vi "configure resonance.vi"(6 "x resonant zoom voltage":dbl, 8 "error in":errorcluster, 10 "Start Delay (Ticks)":i16) -> (0 "bitfile name":T1, 1 "pixels per frame":dbl, 2 "FPGA VI Reference Out":T2, 4 "Actual Depth 3":u32)   [LabVIEW 2012]
doc: "SciScan 1.0 151216"
uses:
  Custom Controls/FPGA reference typedef for 120MHz code.ctl
  Custom Controls/biotfile select.ctl
  Custom Controls/Pockels data structure (for laser power control).ctl
  <vilib>/DAQmx/write.llb/DAQmx Write (Analog DBL 1Chan 1Samp).vi
  <vilib>/DAQmx/write.llb/DAQmx Write (Analog 2D DBL NChan NSamp).vi
  <vilib>/DAQmx/write.llb/DAQmx Write (Analog 1D DBL 1Chan NSamp).vi
  GFG/GFGstringGet.vi
  GFG/GFGbooleanGet.vi
  <vilib>/DAQmx/create/channels.llb/DAQmx Create Channel (AO-Voltage-Basic).vi
  <vilib>/DAQmx/miscellaneous.llb/DAQmx Fill In Error Info.vi
  GFG/GFGnumericGet.vi
  <vilib>/DAQmx/configure/trigger.llb/DAQmx Start Trigger (Digital Edge).vi
  <vilib>/Utility/error.llb/Error Cluster From Error Code.vi
  <vilib>/rvi/errors/niLvFpgaAdjustHostInterfaceError.vi
  <vilib>/rvi/interface/nirviMethod/nirviMethod.xnode
  GFG/GFG library.lvlib
  <resource>/objmgr/daqmx.rc
  <vilib>/rvi/errors/niLvFpgaMergeErrorWithErrorCode.vi
  <vilib>/FPGAPlugInAG/Dynamic/niLvFpga_ReadFifo_Dynamic.vi
panel:
  out "size(s)":i32[](array[numeric])
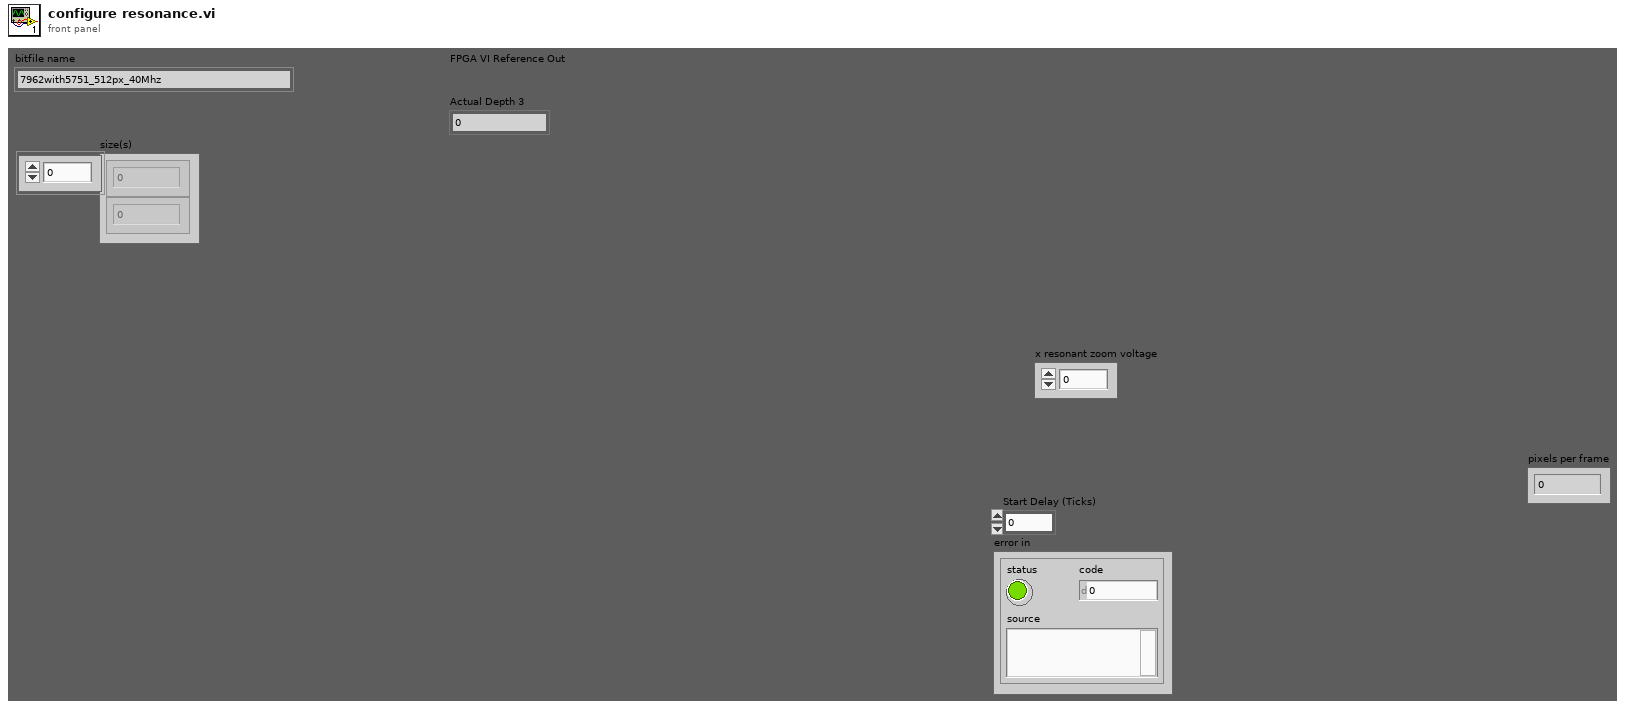
[diagram p1: front panel]
types:
  T1 = typedef "biotfile select.ctl" = enum16{"7962with5751_512px_40Mhz", "7962with5751_512px_50Mhz", "7961with5734_1024px_120Mhz or ext lasersync", "7962with5734_1024px_120Mhz or ext lasersync", "7962with5734_512px_120Mhz or ext lasersync", "7961with5734_512px_120Mhz or ext lasersync", "7962with5751_12kHz_512px_50MHz_4ch", "7962with5751_1536px_2ch_40Mhz", "7962with5751_1536px_2ch_50Mhz", "7962with5751_12kHz_1024px_2ch_50MHz"}
  T2 = typedef "FPGA reference typedef for 120MHz code.ctl" = refnum<k20>
  T3 = typedef "Pockels data structure (for laser power control).ctl" = cluster{"DAQmx Task Name (Pockels)":refnum<k21>, "(Sharing Pocekls Card?)YGalvo, Pockels,Piezo":bool[]}
  T4 = cluster{"bitfile name":T1, dbl, "lasersync enable":bool}
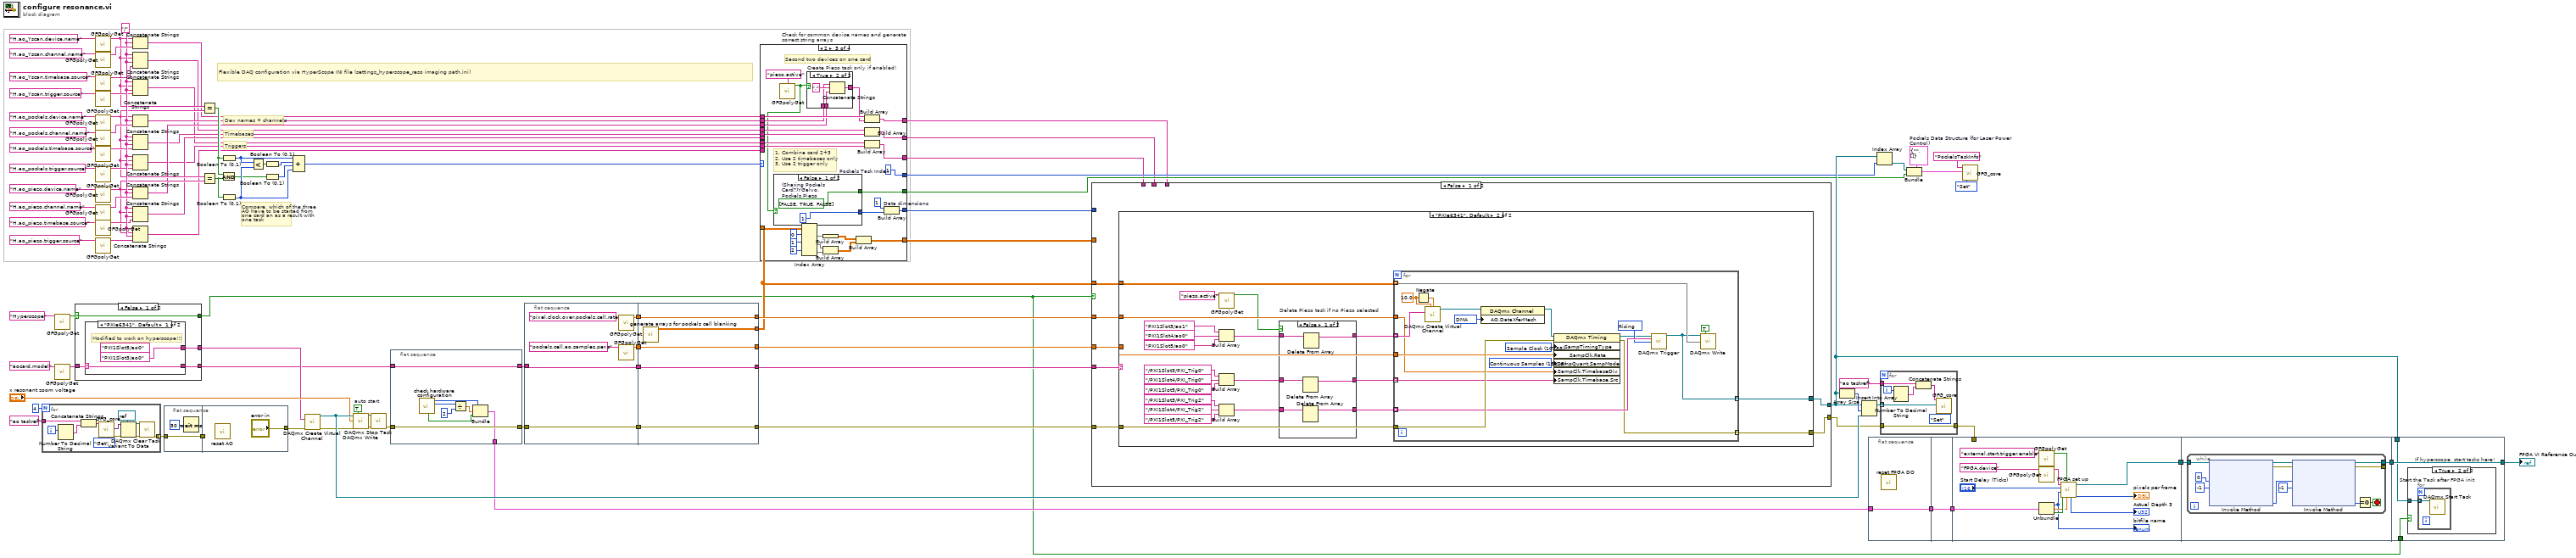
[diagram p0: block diagram]
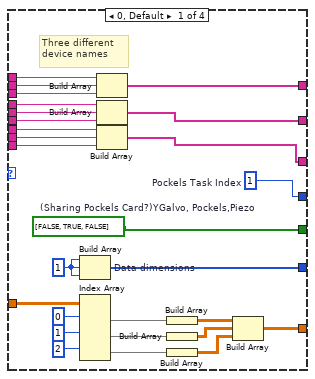
[diagram p2: hidden frame]
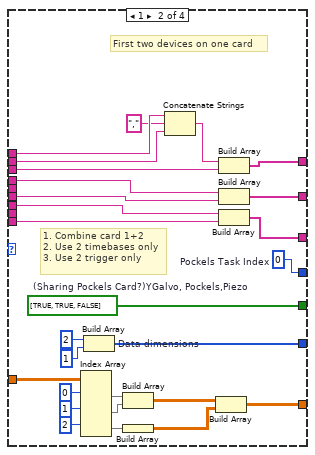
[diagram p3: hidden frame]
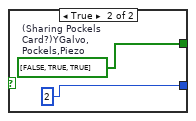
[diagram p4: hidden frame]
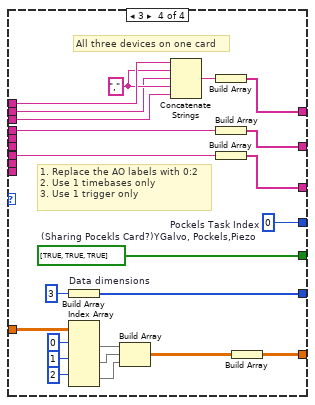
[diagram p6: hidden frame]
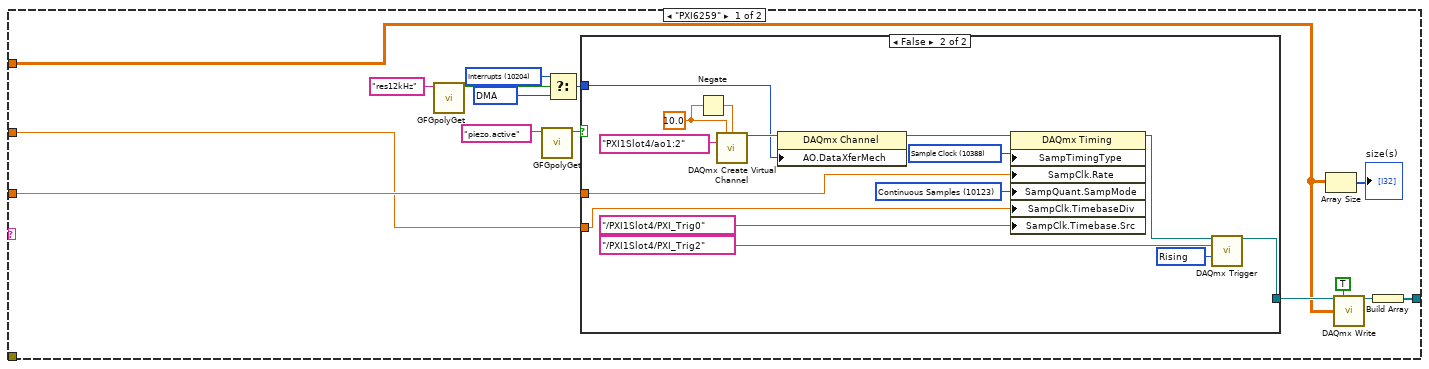
[diagram p7: hidden frame]
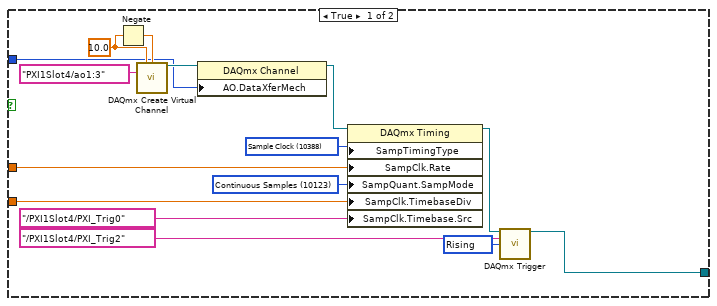
[diagram p8: hidden frame]
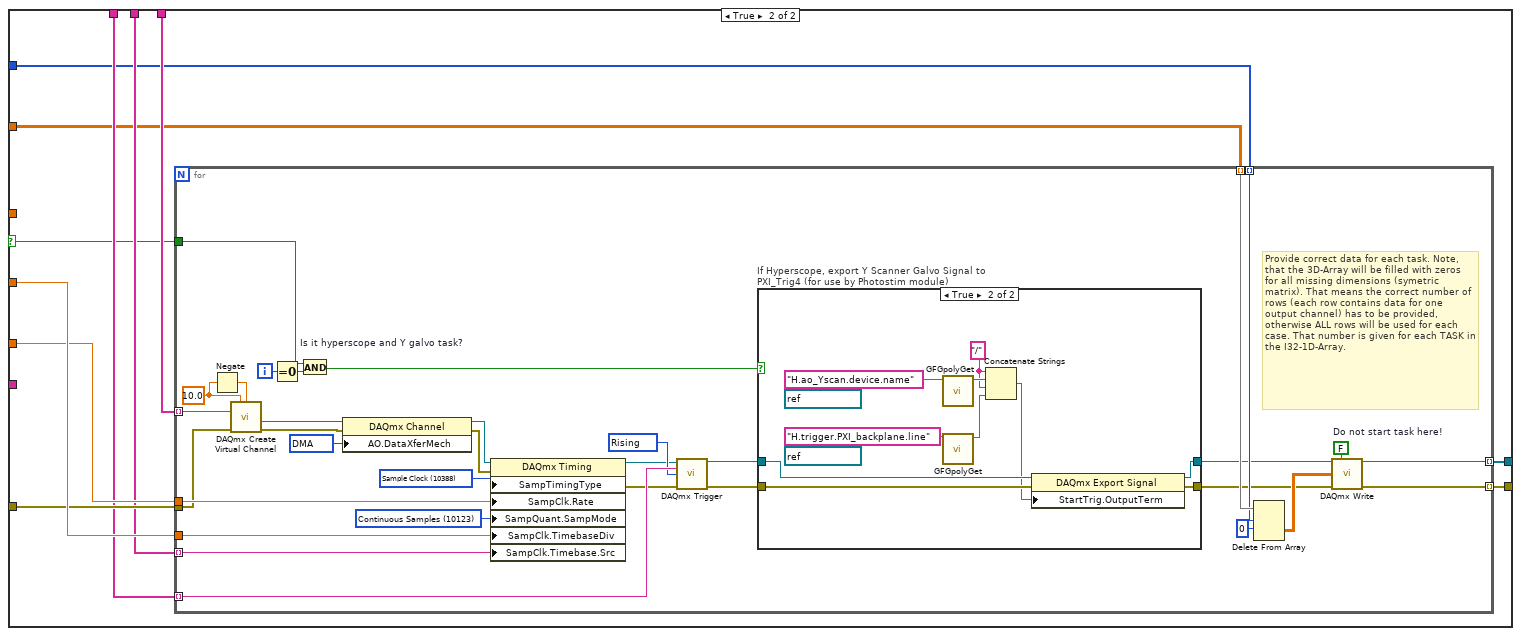
[diagram p10: hidden frame]
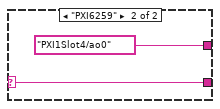
[diagram p12: hidden frame]
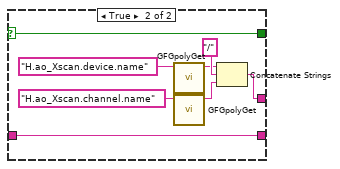
[diagram p13: hidden frame]
diagram:
  w10 = T3 {"DAQmx Task Name (Pockels)"="", "(Sharing Pocekls Card?)YGalvo, Pockels,Piezo"=[]}  # Pockels Data Structure (for Laser Power Control)
  w55 = "/" ("string")
  w91 = TRUE  # auto start
  # "Flexible DAQ configuration via HyperScope INI file (settings_hyperscope_reso imaging path.ini)"
  # "Triggers"
  # "Timebases"
  # "Dev names + channels"
  # "Compare, which of the three AO have to be started from one card an as a result with one task"
  n1 = for {
    N: 4 -> [_]
    tunnel: "ao taskref" ("Variable Name in") -> [w105]
    tunnel: [w100] -> w67 mode=indexing
    i -> [w107]
    n2 = Number To Decimal String(number=w107) -> (decimal integer string=w106:string)  [unwired: 1 in]
    n3 = Concatenate Strings(w105, w106) -> (w104:string)
    n4 = call "GFG_core.vi"("Variable Name in"=w104, "Action"=enum16{"Init", "Set", "Get"}."Get") -> ("Variant Out"=w102:variant, "error out"=w103:errorcluster)  [unwired: 11 in, 5 out]
    n5 = Variant To Data(error in=w103, type=refnum<k21> refnum ("task out"), Variant=w102) -> (data=w99:refnum<k21>, error out=w98:errorcluster)
    n6 = call <vilib>:"DAQmx Clear Task.vi"("task in"=w99, "error in"=w98) -> ("error out"=w100:errorcluster)  [unwired: 13 in]
  }
  n7 = call-poly "GFGpolyGet.vi"("Variable Name in"="aocard.model") -> ("String"=w14:string)  [unwired: 9 in, 1 out]
  n8 = call-poly "GFGpolyGet.vi"("Variable Name in"="Hyperscope") -> ("Boolean Value OUT"=w15:bool)  [unwired: 9 in, 1 out]
  n9 = case shown="False" w15 {
    selector: w15 -> [w110 w118]
    tunnel: [w112 w121] -> w72
    tunnel: w14 -> [w111 w117]
    tunnel: [w110 w118] -> w4
    tunnel: [w109 w117] -> w13
    frame False {
      n10 = case shown="\"PXIe6341\", Default" w111 {
        selector: w111 -> [w114 w115]
        tunnel: [tag "PXI1Slot3/ao0" ("physical channels") tag "PXI1Slot4/ao0" ("physical channels")] -> w112
        tunnel: [w114 w115] -> w109
        frame "PXIe6341", Default {
          (unwired) tag "PXI1Slot5/ao0" ("physical channels")
          # "Modified to work on hyperscope!!!"
        }
        frame "PXI6259" {
        }
      }
    }
    frame True {
      n11 = call-poly "GFGpolyGet.vi"("Variable Name in"="H.ao_Xscan.device.name") -> ("String"=w119:string)  [unwired: 9 in, 1 out]
      n12 = call-poly "GFGpolyGet.vi"("Variable Name in"="H.ao_Xscan.channel.name") -> ("String"=w122:string)  [unwired: 9 in, 1 out]
      n13 = Concatenate Strings(w119, "/" ("String_Output"), w122) -> (w121:string)
    }
  }
  n14 = call-poly "GFGpolyGet.vi"("Variable Name in"="H.ao_Yscan.device.name") -> ("String"=w42:string)  [unwired: 9 in, 1 out]
  n15 = call-poly "GFGpolyGet.vi"("Variable Name in"="H.ao_Yscan.channel.name") -> ("String"=w58:string)  [unwired: 9 in, 1 out]
  n16 = call-poly "GFGpolyGet.vi"("Variable Name in"="H.ao_Yscan.timebase.source") -> ("String"=w52:string)  [unwired: 9 in, 1 out]
  n17 = call-poly "GFGpolyGet.vi"("Variable Name in"="H.ao_Yscan.trigger.source") -> ("String"=w51:string)  [unwired: 9 in, 1 out]
  n18 = call-poly "GFGpolyGet.vi"("Variable Name in"="H.ao_pockels.device.name") -> ("String"=w40:string)  [unwired: 9 in, 1 out]
  n19 = call-poly "GFGpolyGet.vi"("Variable Name in"="H.ao_pockels.channel.name") -> ("String"=w57:string)  [unwired: 9 in, 1 out]
  n20 = call-poly "GFGpolyGet.vi"("Variable Name in"="H.ao_pockels.timebase.source") -> ("String"=w46:string)  [unwired: 9 in, 1 out]
  n21 = call-poly "GFGpolyGet.vi"("Variable Name in"="H.ao_pockels.trigger.source") -> ("String"=w45:string)  [unwired: 9 in, 1 out]
  n22 = call-poly "GFGpolyGet.vi"("Variable Name in"="H.ao_piezo.device.name") -> ("String"=w41:string)  [unwired: 9 in, 1 out]
  n23 = call-poly "GFGpolyGet.vi"("Variable Name in"="H.ao_piezo.channel.name") -> ("String"=w56:string)  [unwired: 9 in, 1 out]
  n24 = call-poly "GFGpolyGet.vi"("Variable Name in"="H.ao_piezo.timebase.source") -> ("String"=w44:string)  [unwired: 9 in, 1 out]
  n25 = call-poly "GFGpolyGet.vi"("Variable Name in"="H.ao_piezo.trigger.source") -> ("String"=w43:string)  [unwired: 9 in, 1 out]
  n26 = Concatenate Strings(w42, w55, w58) -> (w31:string)
  n27 = Concatenate Strings(w55, w42, w55, w52) -> (w28:string)
  n28 = Concatenate Strings(w55, w42, w55, w51) -> (w25:string)
  n29 = Concatenate Strings(w40, w55, w57) -> (w30:string)
  n30 = Concatenate Strings(w55, w40, w55, w46) -> (w27:string)
  n31 = Concatenate Strings(w55, w40, w55, w45) -> (w24:string)
  n32 = Concatenate Strings(w41, w55, w56) -> (w29:string)
  n33 = Concatenate Strings(w55, w41, w55, w44) -> (w26:string)
  n34 = Concatenate Strings(w55, w41, w55, w43) -> (w23:string)
  n35 = flat-sequence {
    tunnel: w67 -> [w126]
    tunnel: [w126] -> w66
    tunnel: ["error in"] -> w74
    tunnel: w66 -> [_]
    frame #0 {
      n36 = Wait (ms)(milliseconds to wait=u32 50) -> ()  [unwired: 1 out]
    }
    frame #1 {
      n37 = call "reset AO.vi"() -> ()  [unwired: 12 in]
    }
  }
  n38 = Equal?(x=w42, y=w40) -> (x = y?=w33:bool)
  n39 = Equal?(x=w40, y=w41) -> (x = y?=w32:bool)
  n40 = Boolean To (0,1)(Boolean=w33) -> (0, 1=w36:i16)
  n41 = And(x=w33, y=w32) -> (x .and. y?=w37:bool)
  n42 = Boolean To (0,1)(Boolean=w32) -> (0, 1=w39:i16)
  n43 = Less?(x=w36, y=w39) -> (x < y?=w34:bool)
  n44 = Boolean To (0,1)(Boolean=w34) -> (0, 1=w35:i16)
  n45 = Boolean To (0,1)(Boolean=w37) -> (0, 1=w38:i16)
  n46 = Compound Arithmetic op=ADD(w36, w35, w38, w39) -> (w22:i16)
  n47 = call-poly <vilib>:"DAQmx Create Virtual Channel.vi"("physical channels"=w72, "error in"=w74) -> ("task out"=w92:refnum<k21>, "error out"=w90:errorcluster)  [unwired: 12 in]
  n48 = call-poly <vilib>:"DAQmx Write.vi"("task/channels in"=w92, "auto start"=w91, "data"="x resonant zoom voltage", "error in"=w90) -> ("task out"=w93:refnum<k21>, "error out"=w88:errorcluster)  [unwired: 9 in, 1 out]
  n49 = call <vilib>:"DAQmx Stop Task.vi"("task/channels in"=w93, "error in"=w88) -> ("error out"=w81:errorcluster)  [unwired: 12 in, 1 out]
  n50 = flat-sequence {
    tunnel: [w133] -> w82
    tunnel: w81 -> [w133]
    tunnel: [w130] -> w79
    tunnel: w13 -> [w128]
    tunnel: [w128] -> w71
    frame #0 {
      n51 = call "check hardware configuration.vi"() -> ("number of lines"=w134:i32, "bitfile name"=w131:T1, "lasersync enable"=w132:bool)  [unwired: 7 in, 2 out]
      n52 = Divide(x=w134, y=2) -> (x/y=w129:dbl)
      n53 = Bundle("bitfile name"=w131, w129, "lasersync enable"=w132) -> (w130:T4)  [unwired: 1 in]
    }
  }
  n54 = flat-sequence {
    tunnel: [w140] -> w85
    tunnel: [w136] -> w84
    tunnel: [w138] -> w83
    tunnel: w82 -> [w137]
    tunnel: [w137] -> w76
    tunnel: w71 -> [w136]
    tunnel: [w144] -> w86
    tunnel: [w145] -> w87
    tunnel: [w146] -> w97
    tunnel: w85 -> [w146]
    tunnel: w84 -> [w145]
    tunnel: w83 -> [w144]
    tunnel: [w143] -> w19
    tunnel: [w142] -> w75
    tunnel: w76 -> [w142]
    frame #0 {
      n55 = call-poly "GFGpolyGet.vi"("Variable Name in"="pixel.clock.over.pockels.cell.rate") -> ("Numeric"=w138:dbl)  [unwired: 8 in, 2 out]
      n56 = call-poly "GFGpolyGet.vi"("Variable Name in"="pockels.cell.ao.samples.per.s") -> ("Numeric"=w140:dbl)  [unwired: 8 in, 2 out]
    }
    frame #1 {
      n57 = call "generate arrays for pockels cell blanking.vi"() -> ("Array"=w143:dbl[][])  [unwired: 11 in]
    }
  }
  n58 = case "Check for common device names and generate correct string arrays" shown="2" w22 {
    tunnel: [w149 w200 w227 w259] -> w1
    tunnel: w31 -> [w173 w183 w228 w246]
    tunnel: w30 -> [w172 w182 w209 w244]
    tunnel: w29 -> [w171 w199 w208 w243]
    tunnel: w28 -> [w170 w194 w226 w258]
    tunnel: w27 -> [w166 _ w225 _]
    tunnel: w26 -> [w169 w198 _ _]
    tunnel: [w147 w197 w222 w256] -> w2
    tunnel: w25 -> [w168 w193 w224 w257]
    tunnel: w24 -> [w165 _ w223 _]
    tunnel: w23 -> [w167 w196 _ _]
    tunnel: [w148 w195 w221 w255] -> w3
    tunnel: w19 -> [w164 w190 w220 w254]
    tunnel: [w160 w188 w219 w251] -> w21
    tunnel: [w159 w187 w217 w250] -> w20
    tunnel: [w151 w176 w204 w239] -> w7
    tunnel: [w150 w175 w201 w238] -> w6
    frame 0, Default {
      w150 = bool[] [FALSE, TRUE, FALSE]  # (Sharing Pockels Card?)YGalvo, Pockels,Piezo
      w151 = 1  # Pockels Task Index
      w155 = 1
      # "Three different device names"
      n59 = Build Array "Data dimensions"(w155, w155, w155) -> (w159:i32[])
      n60 = Index Array(array=w164, index (row) #1=0 ("disabled index (col)"), index (row) #2=1 ("index (col)"), index (row) #3=2 ("index (col)")) -> (element #1=w163:dbl[], element #2=w153:dbl[], element #3=w154:dbl[])  [unwired: 3 in]
      n61 = Build Array(w173, w172, w171) -> (w149:string[])
      n62 = Build Array(w170, w166, w169) -> (w147:string[])
      n63 = Build Array(w168, w165, w167) -> (w148:string[])
      n64 = Build Array(w163) -> (w162:dbl[][])
      n65 = Build Array(w153) -> (w152:dbl[][])
      n66 = Build Array(w154) -> (w161:dbl[][])
      n67 = Build Array(w162, w152, w161) -> (w160:dbl[][][])
    }
    frame 1 {
      w175 = bool[] [TRUE, TRUE, FALSE]  # (Sharing Pockels Card?)YGalvo, Pockels,Piezo
      w176 = 0  # Pockels Task Index
      # "1. Combine card 1+2\n2. Use 2 timebases only\n3. Use 2 trigger only"
      # "First two devices on one card"
      n68 = Index Array(array=w190, index (row) #1=0 ("disabled index (col)"), index (row) #2=1 ("index (col)"), index (row) #3=2 ("index (col)")) -> (element #1=w192:dbl[], element #2=w189:dbl[], element #3=w191:dbl[])  [unwired: 3 in]
      n69 = Build Array "Data dimensions"(2, 1) -> (w187:i32[])
      n70 = Build Array(w192, w189) -> (w177:dbl[][])
      n71 = Build Array(w191) -> (w180:dbl[][])
      n72 = Concatenate Strings(w183, ",", w182) -> (w181:string)
      n73 = Build Array(w177, w180) -> (w188:dbl[][][])
      n74 = Build Array(w181, w199) -> (w200:string[])
      n75 = Build Array(w194, w198) -> (w197:string[])
      n76 = Build Array(w193, w196) -> (w195:string[])
    }
    frame 2 {
      w204 = 1  # Pockels Task Index
      # "1. Combine card 2+3\n2. Use 2 timebases only\n3. Use 2 trigger only"
      # "Second two devices on one card"
      n77 = call-poly "GFGpolyGet.vi"("Variable Name in"="piezo.active") -> ("Boolean Value OUT"=w202:bool)  [unwired: 9 in, 1 out]
      n78 = case shown="False" w202 {
        tunnel: [1 2] -> w206
        tunnel: [w229 w231] -> w201
        frame False {
          w229 = bool[] [FALSE, TRUE, FALSE]  # (Sharing Pockels Card?)YGalvo, Pockels,Piezo
        }
        frame True {
          w231 = bool[] [FALSE, TRUE, TRUE]  # (Sharing Pockels Card?)YGalvo, Pockels,Piezo
        }
      }
      n79 = Index Array(array=w220, index (row) #1=0 ("disabled index (col)"), index (row) #2=1 ("index (col)"), index (row) #3=2 ("index (col)")) -> (element #1=w216:dbl[], element #2=w213:dbl[], element #3=w215:dbl[])  [unwired: 3 in]
      n80 = case "Create Piezo task only if enabled!" shown="True" w202 {
        tunnel: w209 -> [w233 w236]
        tunnel: w208 -> [_ w235]
        tunnel: [w233 w234] -> w207
        frame False {
        }
        frame True {
          n81 = Concatenate Strings(w236, ",", w235) -> (w234:string)
        }
      }
      n82 = Build Array(w216) -> (w214:dbl[][])
      n83 = Build Array(w213, w215) -> (w205:dbl[][])
      n84 = Build Array(w214, w205) -> (w219:dbl[][][])
      n85 = Build Array(w228, w207) -> (w227:string[])
      n86 = Build Array(w226, w225) -> (w222:string[])
      n87 = Build Array(w224, w223) -> (w221:string[])
      n88 = Build Array "Data dimensions"(1, w206) -> (w217:i32[])
    }
    frame 3 {
      w238 = bool[] [TRUE, TRUE, TRUE]  # (Sharing Pocekls Card?)YGalvo, Pockels,Piezo
      w239 = 0  # Pockels Task Index
      w245 = ","
      # "1. Replace the AO labels with 0:2\n2. Use 1 timebases only\n3. Use 1 trigger only"
      # "All three devices on one card"
      n89 = Build Array "Data dimensions"(3) -> (w250:i32[])
      n90 = Index Array(array=w254, index (row) #1=0 ("disabled index (col)"), index (row) #2=1 ("index (col)"), index (row) #3=2 ("index (col)")) -> (element #1=w253:dbl[], element #2=w252:dbl[], element #3=w242:dbl[])  [unwired: 3 in]
      n91 = Build Array(w253, w252, w242) -> (w240:dbl[][])
      n92 = Concatenate Strings(w246, w245, w244, w245, w243) -> (w260:string)
      n93 = Build Array(w260) -> (w259:string[])
      n94 = Build Array(w258) -> (w256:string[])
      n95 = Build Array(w257) -> (w255:string[])
      n96 = Build Array(w240) -> (w251:dbl[][][])
    }
  }
  n97 = case shown="False" w4 {
    selector: w4 -> [_ w364]
    tunnel: w97 -> [w267 w373]
    tunnel: [w266 w371] -> w8
    tunnel: w87 -> [w265 _]
    tunnel: w86 -> [w264 w374]
    tunnel: [w263 w370] -> w80
    tunnel: w75 -> [w262 w372]
    tunnel: w1 -> [_ w369]
    tunnel: w2 -> [_ w368]
    tunnel: w3 -> [_ w367]
    tunnel: w21 -> [_ w366]
    tunnel: w20 -> [_ w365]
    tunnel: w19 -> [w261 _]
    frame False {
      n98 = case shown="\"PXIe6341\", Default" w265 {
        tunnel: w267 -> [w279 w335]
        tunnel: w261 -> [w275 w334]
        tunnel: [w276 w325] -> w266
        tunnel: w262 -> [_ w324]
        tunnel: w264 -> [w278 w323]
        tunnel: [_ w322] -> w263
        frame "PXI6259" {
          w269 = 10054 items=["DMA"=10054, "Interrupts"=10204, "Programmed I/O"=10264, "USB Bulk"=12590] ("AO.DataXferMech")
          w270 = 10204 items=["DMA"=10054, "Interrupts"=10204, "Programmed I/O"=10264, "USB Bulk"=12590] ("AO.DataXferMech")
          n99 = call-poly "GFGpolyGet.vi"("Variable Name in"="res12kHz") -> ("Boolean Value OUT"=w271:bool)  [unwired: 9 in, 1 out]
          n100 = call-poly "GFGpolyGet.vi"("Variable Name in"="piezo.active") -> ("Boolean Value OUT"=w281:bool)  [unwired: 9 in, 1 out]
          n101 = Select(t=w270, s=w271, f=w269) -> (s? t:f=w268:i32)
          n102 = case shown="False" w281 {
            tunnel: w279 -> [w291 w306]
            tunnel: [w286 w303] -> w282
            tunnel: w278 -> [w290 w305]
            tunnel: w268 -> [w283 w298]
            frame True {
              w289 = 10280 items=["Rising"=10280, "Falling"=10171] ("edge")
              w293 = 10388 items=["Sample Clock"=10388, "Burst Handshake"=12548, "Handshake"=10389, "Implicit"=10451, "On Demand"=10390, "Change Detection"=12504, "Pipelined Sample Clock"=14668] ("SampTimingType")
              w294 = 10123 items=["Finite Samples"=10178, "Continuous Samples"=10123, "Hardware Timed Single Point"=12522] ("SampQuant.SampMode")
              w296 = 10.0 ("maximum value")
              n103 = Negate(x=w296) -> (-x=w297:dbl)
              n104 = call-poly <vilib>:"DAQmx Create Virtual Channel.vi"("maximum value"=w296, "minimum value"=w297, "physical channels"=tag "PXI1Slot4/ao1:3") -> ("task out"=w284:refnum<k21>)  [unwired: 11 in, 1 out]
              n105 = property class="DAQmx Channel"(reference=w284, "AO.DataXferMech"=w283) -> (reference out=w285:refnum<k21>)  [unwired: 1 in, 1 out]
              n106 = property class="DAQmx Timing"(reference=w285, "SampTimingType"=w293, "SampClk.Rate"=w291, "SampQuant.SampMode"=w294, "SampClk.TimebaseDiv"=w290, "SampClk.Timebase.Src"=tag "/PXI1Slot4/PXI_Trig0" ("SampClk.Src")) -> (reference out=w287:refnum<k21>)  [unwired: 1 in, 1 out]
              n107 = call-poly <vilib>:"DAQmx Trigger.vi"("task/channels in"=w287, "source"=tag "/PXI1Slot4/PXI_Trig2", "edge"=w289) -> ("task out"=w286:refnum<k21>)  [unwired: 11 in, 1 out]
            }
            frame False {
              w302 = 10280 items=["Rising"=10280, "Falling"=10171] ("edge")
              w308 = 10388 items=["Sample Clock"=10388, "Burst Handshake"=12548, "Handshake"=10389, "Implicit"=10451, "On Demand"=10390, "Change Detection"=12504, "Pipelined Sample Clock"=14668] ("SampTimingType")
              w309 = 10123 items=["Finite Samples"=10178, "Continuous Samples"=10123, "Hardware Timed Single Point"=12522] ("SampQuant.SampMode")
              w311 = 10.0 ("maximum value")
              n108 = Negate(x=w311) -> (-x=w312:dbl)
              n109 = call-poly <vilib>:"DAQmx Create Virtual Channel.vi"("maximum value"=w311, "minimum value"=w312, "physical channels"=tag "PXI1Slot4/ao1:2") -> ("task out"=w300:refnum<k21>)  [unwired: 11 in, 1 out]
              n110 = property class="DAQmx Channel"(reference=w300, "AO.DataXferMech"=w298) -> (reference out=w299:refnum<k21>)  [unwired: 1 in, 1 out]
              n111 = property class="DAQmx Timing"(reference=w299, "SampTimingType"=w308, "SampClk.Rate"=w306, "SampQuant.SampMode"=w309, "SampClk.TimebaseDiv"=w305, "SampClk.Timebase.Src"=tag "/PXI1Slot4/PXI_Trig0" ("SampClk.Src")) -> (reference out=w304:refnum<k21>)  [unwired: 1 in, 1 out]
              n112 = call-poly <vilib>:"DAQmx Trigger.vi"("task/channels in"=w304, "source"=tag "/PXI1Slot4/PXI_Trig2", "edge"=w302) -> ("task out"=w303:refnum<k21>)  [unwired: 11 in, 1 out]
            }
          }
          n113 = Array Size(array=w275) -> (size(s)=→"size(s)":i32[])
          n114 = call-poly <vilib>:"DAQmx Write.vi"("task/channels in"=w282, "auto start"=TRUE, "data"=w275) -> ("task out"=w277:refnum<k21>)  [unwired: 10 in, 2 out]
          n115 = Build Array(w277) -> (w276:refnum<k21>[])
        }
        frame "PXIe6341", Default {
          n116 = Build Array(tag "PXI1Slot3/ao1" ("physical channels"), tag "PXI1Slot4/ao0" ("physical channels"), tag "PXI1Slot5/ao0" ("physical channels")) -> (w319:tag[])
          n117 = Build Array(tag "/PXI1Slot3/PXI_Trig0" ("SampClk.Src"), tag "/PXI1Slot4/PXI_Trig0" ("SampClk.Src"), tag "/PXI1Slot5/PXI_Trig0" ("SampClk.Src")) -> (w318:tag[])
          n118 = Build Array(tag "/PXI1Slot3/PXI_Trig2" ("source"), tag "/PXI1Slot4/PXI_Trig2" ("source"), tag "/PXI1Slot5/PXI_Trig2" ("source")) -> (w317:tag[])
          n119 = call-poly "GFGpolyGet.vi"("Variable Name in"="piezo.active") -> ("Boolean Value OUT"=w313:bool)  [unwired: 9 in, 1 out]
          n120 = case "Delete Piezo task if no Piezo selected" shown="False" w313 {
            tunnel: w319 -> [w337 w342]
            tunnel: w318 -> [w339 w343]
            tunnel: w317 -> [w341 w344]
            tunnel: [w340 w344] -> w316
            tunnel: [w338 w343] -> w315
            tunnel: [w336 w342] -> w314
            frame False {
              n121 = Delete From Array(array=w339) -> (array with subset deleted=w338:tag[])  [unwired: 2 in, 1 out]
              n122 = Delete From Array(array=w341) -> (array with subset deleted=w340:tag[])  [unwired: 2 in, 1 out]
              n123 = Delete From Array(array=w337) -> (array with subset deleted=w336:tag[])  [unwired: 2 in, 1 out]
            }
            frame True {
            }
          }
          n124 = for {
            tunnel: w323 -> [w354]
            tunnel: [w352] -> w325 mode=indexing
            tunnel: w324 -> [w359]
            tunnel: w314 -> [w363] mode=indexing
            tunnel: w335 -> [w355]
            tunnel: w334 -> [w358] mode=indexing
            tunnel: w316 -> [w353] mode=indexing
            tunnel: w315 -> [w356] mode=indexing
            tunnel: [w346] -> w322 mode=indexing
            w345 = 10054 items=["DMA"=10054, "Interrupts"=10204, "Programmed I/O"=10264, "USB Bulk"=12590] ("AO.DataXferMech")
            w348 = 10280 items=["Rising"=10280, "Falling"=10171] ("edge")
            w350 = 10388 items=["Sample Clock"=10388, "Burst Handshake"=12548, "Handshake"=10389, "Implicit"=10451, "On Demand"=10390, "Change Detection"=12504, "Pipelined Sample Clock"=14668] ("SampTimingType")
            w351 = 10123 items=["Finite Samples"=10178, "Continuous Samples"=10123, "Hardware Timed Single Point"=12522] ("SampQuant.SampMode")
            w361 = 10.0 ("maximum value")
            n125 = Negate(x=w361) -> (-x=w362:dbl)
            n126 = call-poly <vilib>:"DAQmx Create Virtual Channel.vi"("maximum value"=w361, "minimum value"=w362, "physical channels"=w363) -> ("task out"=w357:refnum<k21>)  [unwired: 11 in, 1 out]
            n127 = property class="DAQmx Channel"(reference=w357, "AO.DataXferMech"=w345) -> (reference out=w349:refnum<k21>)  [unwired: 1 in, 1 out]
            n128 = property class="DAQmx Timing"(reference=w349, error in=w359, "SampTimingType"=w350, "SampClk.Rate"=w355, "SampQuant.SampMode"=w351, "SampClk.TimebaseDiv"=w354, "SampClk.Timebase.Src"=w356) -> (reference out=w347:refnum<k21>, error out=w346:errorcluster)
            n129 = call-poly <vilib>:"DAQmx Trigger.vi"("task/channels in"=w347, "source"=w353, "edge"=w348) -> ("task out"=w352:refnum<k21>)  [unwired: 11 in, 1 out]
            n130 = call-poly <vilib>:"DAQmx Write.vi"("task/channels in"=w352, "auto start"=TRUE, "data"=w358) -> ()  [unwired: 10 in, 3 out]
          }
        }
      }
    }
    frame True {
      n131 = for {
        tunnel: w374 -> [w401]
        tunnel: [w377] -> w371 mode=indexing
        tunnel: w372 -> [w390]
        tunnel: w369 -> [w407] mode=indexing
        tunnel: w373 -> [w402]
        tunnel: w367 -> [w400] mode=indexing
        tunnel: w368 -> [w403] mode=indexing
        tunnel: [w379] -> w370 mode=indexing
        tunnel: w366 -> [w389] mode=indexing
        tunnel: w365 -> [w388] mode=indexing
        tunnel: w364 -> [w375]
        i -> [w384]
        w376 = FALSE  # Do not start task here!
        w394 = 10054 items=["DMA"=10054, "Interrupts"=10204, "Programmed I/O"=10264, "USB Bulk"=12590] ("AO.DataXferMech")
        w396 = 10280 items=["Rising"=10280, "Falling"=10171] ("edge")
        w398 = 10388 items=["Sample Clock"=10388, "Burst Handshake"=12548, "Handshake"=10389, "Implicit"=10451, "On Demand"=10390, "Change Detection"=12504, "Pipelined Sample Clock"=14668] ("SampTimingType")
        w399 = 10123 items=["Finite Samples"=10178, "Continuous Samples"=10123, "Hardware Timed Single Point"=12522] ("SampQuant.SampMode")
        w405 = 10.0 ("maximum value")
        # "Provide correct data for each task. Note, that the 3D-Array will be filled with zeros for all missing dimensions (symetric matrix). That means the correct number of rows (each row contains data for one output channel) has to be provided, otherwise ALL rows will be used for each case. That number is given for each TASK in the I32-1D-Array."
        n132 = Negate(x=w405) -> (-x=w406:dbl)
        n133 = call-poly <vilib>:"DAQmx Create Virtual Channel.vi"("maximum value"=w405, "minimum value"=w406, "physical channels"=w407, "error in"=w390) -> ("task out"=w404:refnum<k21>, "error out"=w392:errorcluster)  [unwired: 10 in]
        n134 = Equal To 0?(x=w384) -> (x = 0?=w383:bool)
        n135 = And "Is it hyperscope and Y galvo task?"(x=w375, y=w383) -> (x .and. y?=w385:bool)
        n136 = property class="DAQmx Channel"(reference=w404, error in=w392, "AO.DataXferMech"=w394) -> (reference out=w397:refnum<k21>, error out=w391:errorcluster)
        n137 = property class="DAQmx Timing"(reference=w397, error in=w391, "SampTimingType"=w398, "SampClk.Rate"=w402, "SampQuant.SampMode"=w399, "SampClk.TimebaseDiv"=w401, "SampClk.Timebase.Src"=w403) -> (reference out=w395:refnum<k21>, error out=w393:errorcluster)
        n138 = call-poly <vilib>:"DAQmx Trigger.vi"("task/channels in"=w395, "source"=w400, "edge"=w396, "error in"=w393) -> ("task out"=w382:refnum<k21>, "error out"=w381:errorcluster)  [unwired: 10 in]
        n139 = case "If Hyperscope, export Y Scanner Galvo Signal to PXI_Trig4 (for use by Photostim module)" shown="True" w385 {
          tunnel: w382 -> [w409 w419]
          tunnel: [w409 w416] -> w378
          tunnel: w381 -> [w408 w418]
          tunnel: [w408 w417] -> w380
          frame False {
          }
          frame True {
            (unwired) refnum<k21> "PXI_Trig4" ("task out")
            (unwired) refnum<k21> "PXI1Slot3" ("task out")
            w412 = "/" ("Variable Name in")
            n140 = call-poly "GFGpolyGet.vi"("Variable Name in"="H.ao_Yscan.device.name") -> ("String"=w414:string)  [unwired: 9 in, 1 out]
            n141 = call-poly "GFGpolyGet.vi"("Variable Name in"="H.trigger.PXI_backplane.line") -> ("String"=w410:string)  [unwired: 9 in, 1 out]
            n142 = Concatenate Strings(w412, w414, w412, w410) -> (w413:string)
            n143 = property class="DAQmx Export Signal"(reference=w419, error in=w418, "StartTrig.OutputTerm"=w413) -> (reference out=w416:refnum<k21>, error out=w417:errorcluster)
          }
        }
        n144 = Delete From Array(array=w389, length=w388, index (row)=0) -> (deleted portion=w387:dbl[][])  [unwired: 1 in, 1 out]
        n145 = call-poly <vilib>:"DAQmx Write.vi"("task/channels in"=w378, "auto start"=w376, "data"=w387, "error in"=w380) -> ("task out"=w377:refnum<k21>, "error out"=w379:errorcluster)  [unwired: 9 in, 1 out]
      }
    }
  }
  n146 = Array Size(array=w8) -> (size(s)=w94:i32)
  n147 = Insert Into Array(array=w8, index=w94, new element=w92) -> (w95:refnum<k21>[])
  n148 = flat-sequence {
    tunnel: [w420] -> w18
    tunnel: w79 -> [w420]
    tunnel: w18 -> [w421]
    tunnel: [w421] -> w17
    tunnel: [w423] -> w77
    tunnel: w17 -> [w426]
    tunnel: w70 -> [_]
    tunnel: w77 -> [w435]
    tunnel: [w434] -> w16
    tunnel: [w449] -> w78
    tunnel: w16 -> [w449]
    tunnel: w8 -> [w448]
    tunnel: w4 -> [w447]
    frame #0 {
      n149 = call "reset FPGA DO.vi"() -> ()  [unwired: 12 in]
    }
    frame #1 {
    }
    frame #2 {
      n150 = call-poly "GFGpolyGet.vi"("Variable Name in"="external.start.trigger.enable") -> ("Boolean Value OUT"=w429:bool)  [unwired: 9 in, 1 out]
      n151 = call-poly "GFGpolyGet.vi"("Variable Name in"="FPGA.device") -> ("String"=w431:string)  [unwired: 9 in, 1 out]
      n152 = Unbundle(w426) -> ("bitfile name"=w422:T1, w424:dbl, "lasersync enable"=w425:bool)
      "bitfile name" <- w422
      n153 = call "FPGA set up.vi"("mirror cycles per frame"=w424, "enable external trigger"=w429, "lasersync"=w425, "bitfile name"=w422, "Start Delay (Ticks)"="Start Delay (Ticks)", "resource name"=w431) -> ("pixels per frame"=→"pixels per frame":i32, "FPGA VI Reference Out"=w423:T2, "Actual Depth 3"=→"Actual Depth 3":u32)  [unwired: 3 in]
    }
    frame #3 {
      n154 = while {
        tunnel: [w445] -> w434
        tunnel: [w444] -> _
        tunnel: w435 -> [w439]
        stop <- w446 stop-if-true
        n155 = xnode "Invoke Method"("FPGA VI Reference In"=w439, "Number of Elements"=u32 0, "Timeout (ms)"=-1) -> ("FPGA VI Reference Out"=w442:T2, "error out"=w441:errorcluster, "Elements Remaining"=w440:u32)  [unwired: 1 in, 1 out]
        n156 = xnode "Invoke Method"("FPGA VI Reference In"=w442, "error in"=w441, "Number of Elements"=w440, "Timeout (ms)"=-1) -> ("FPGA VI Reference Out"=w445:T2, "error out"=w444:errorcluster, "Elements Remaining"=w443:u32)  [unwired: 1 out]
        n157 = Equal To 0?(x=w443) -> (x = 0?=w446:bool)
      }
    }
    frame #4 {
      n158 = case "If hyperscope, start tasks here!" shown="True" w447 {
        tunnel: w448 -> [_ w450]
        frame False {
        }
        frame True {
          n159 = for "Start the Task after FPGA init" {
            tunnel: w450 -> [w451] mode=indexing
            n160 = call <vilib>:"DAQmx Start Task.vi"("task/channels in"=w451) -> ()  [unwired: 13 in, 2 out]
          }
        }
      }
    }
  }
  n161 = Index Array(array=w8, index=w7) -> (element=w5:refnum<k21>)
  n162 = for {
    tunnel: w95 -> [w457] mode=indexing
    tunnel: "ao taskref" ("Variable Name in") -> [w454]
    tunnel: [w452] -> w70
    tunnel: w80 -> [w452]
    i -> [w456]
    n163 = Number To Decimal String(number=w456) -> (decimal integer string=w455:string)  [unwired: 1 in]
    n164 = Concatenate Strings(w454, w455) -> (w453:string)
    n165 = call "GFG_core.vi"("Variable Name in"=w453, "Variant in"=w457, "Action"=enum16{"Init", "Set", "Get"}."Set") -> ()  [unwired: 10 in, 7 out]
  }
  n166 = Bundle(cluster=w10, "DAQmx Task Name (Pockels)"=w5, "(Sharing Pocekls Card?)YGalvo, Pockels,Piezo"=w6) -> (w9:T3)
  n167 = call "GFG_core.vi"("Variable Name in"="PockelsTaskInfo", "Variant in"=w9, "Action"=enum16{"Init", "Set", "Get"}."Set") -> ()  [unwired: 10 in, 7 out]
  "FPGA VI Reference Out" <- w78
